vi "write to fifo.vi"(0 "5785_2_x_1600MHz in":refnum<class "5785_2_x_1600MHz.lvclass">, 11 "error in (no error)":errorcluster) -> (4 "5785_2_x_1600MHz out":refnum<class "5785_2_x_1600MHz.lvclass">, 6 "done write file":bool=TRUE, 8 "num of pulses sent to the FPGA":u32, 10 "room on fifo":bool=TRUE, 15 "error out":errorcluster)   [LabVIEW 2021, in "5785_2_x_1600MHz.lvclass"]
uses:
  5785_2_x_1600MHz.lvclass
  5785_2_x_1600MHz.lvclass/5785_2_x_1600MHz.ctl
  <vilib>/Utility/error.llb/Error Cluster From Error Code.vi
  <vilib>/rvi/errors/niLvFpgaAdjustHostInterfaceError.vi
  <vilib>/rvi/interface/nirviMethod/nirviMethod.xnode
  <vilib>/FPGAPlugInAG/Dynamic/niLvFpga_WriteFifo_Dynamic.vi
  <vilib>/rvi/errors/niLvFpgaMergeErrorWithErrorCode.vi
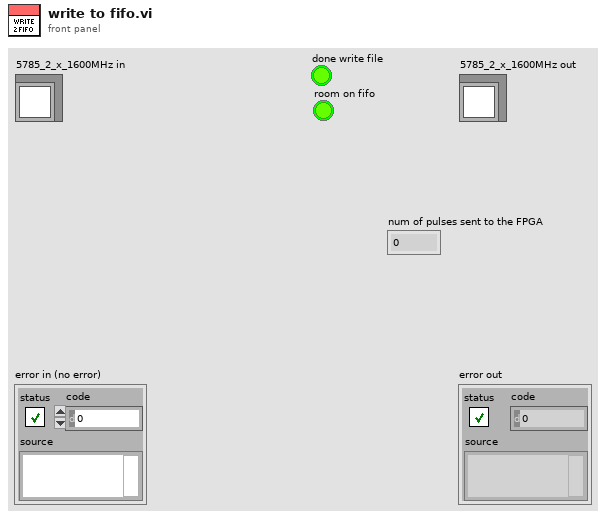
[diagram p1: front panel]
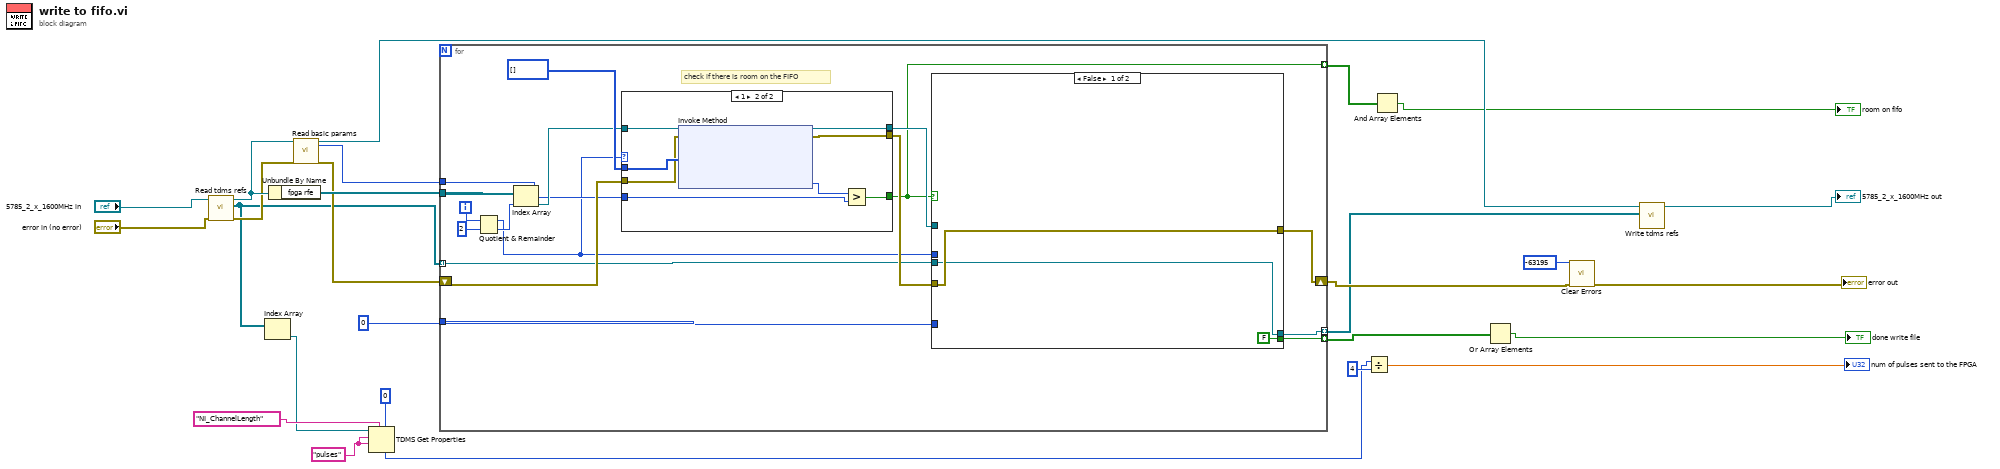
[diagram p0: block diagram]
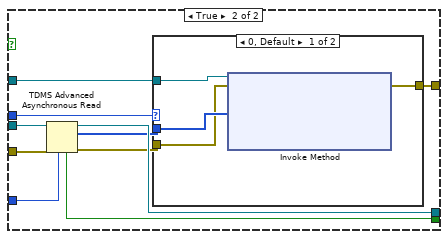
[diagram p2: hidden frame]
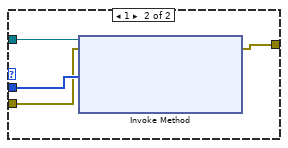
[diagram p3: hidden frame]
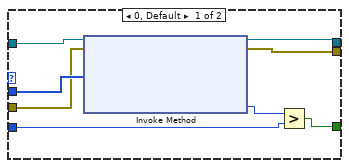
[diagram p4: hidden frame]
diagram:
  w5 = "pulses" ("channel name")
  n1 = call-dynamic "Read tdms refs.vi"("error in (no error)"="error in (no error)", "device_type in"="5785_2_x_1600MHz in") -> ("error out"=w15:errorcluster, "tdms refs"=w3:refnum<k34>[], "device_type out"=w17:refnum<class "5785_2_x_1600MHz.lvclass">)  [unwired: 7 in]
  n2 = Index Array(array=w3) -> (element=w2:refnum<k34>)  [unwired: 1 in]
  n3 = Unbundle By Name(w17) -> ("fpga rfe"=w23:refnum<k20>[])
  n4 = call-dynamic "Read basic params.vi"("device_type in"=w17, "error in (no error)"=w15) -> ("device_type out"=w16:refnum<class "5785_2_x_1600MHz.lvclass">, "buffer size"=w19:u32, "error out"=w14:errorcluster)  [unwired: 12 in, 3 out]
  n5 = TDMS Get Properties(5:u64 0, 7:"NI_ChannelLength" ("property name"), 9:w5, 10:w5, 11:w2) -> (4:w4:u64)  [unwired: 1 in, 5 out]
  n6 = for {
    tunnel: w3 -> [w27] mode=indexing
    tunnel: w23 -> [w43]
    tunnel: u64 0 ("type") -> [w40]
    tunnel: [w39] -> w24 mode=indexing
    tunnel: [w38] -> w18 mode=indexing
    shift-right: [w37] -> w21
    shift-left: w14 -> [w35]
    tunnel: w19 -> [w33]
    tunnel: [w30] -> w20 mode=indexing
    i -> [w28]
    # "check if there is room on the FIFO"
    n7 = Quotient & Remainder(x=w28, y=2) -> (x-y*floor(x/y)=w29:i32, floor(x/y)=w41:i32)
    n8 = Index Array(array=w43, index=w41) -> (element=w34:refnum<k20>)
    n9 = case shown="1" w29 {
      tunnel: w34 -> [w72 w80]
      tunnel: u64[] [] -> [w71 w79]
      tunnel: w35 -> [w70 w78]
      tunnel: [w69 w77] -> w32
      tunnel: w33 -> [w65 w73]
      tunnel: [w67 w75] -> w30
      tunnel: [w66 w74] -> w31
      frame 0, Default {
        n10 = xnode "Invoke Method"("FPGA VI Reference In"=w72, "error in"=w70, "Data"=w71) -> ("FPGA VI Reference Out"=w66:refnum<k20>, "error out"=w69:errorcluster, "Empty Elements Remaining"=w68:u32)  [unwired: 1 in]
        n11 = Greater?(x=w68, y=w65) -> (0:w67:bool)
      }
      frame 1 {
        n12 = xnode "Invoke Method"("FPGA VI Reference In"=w80, "error in"=w78, "Data"=w79) -> ("FPGA VI Reference Out"=w74:refnum<k20>, "error out"=w77:errorcluster, "Empty Elements Remaining"=w76:u32)  [unwired: 1 in]
        n13 = Greater?(x=w76, y=w73) -> (0:w75:bool)
      }
    }
    n14 = case shown="False" w30 {
      tunnel: w27 -> [w44 w47]
      tunnel: w29 -> [_ w56]
      tunnel: w40 -> [_ w55]
      tunnel: [FALSE ("read process finished?") w54] -> w39
      tunnel: [w44 w53] -> w38
      tunnel: [w46 w51] -> w37
      tunnel: w32 -> [w46 w49]
      tunnel: w31 -> [_ w48]
      frame False {
      }
      frame True {
        n15 = TDMS Advanced Asynchronous Read(6:w55, 8:w49, 11:w47) -> (0:w52:errorcluster, 2:w50:u64[], 3:w53:refnum<k34>, 4:w54:bool)
        n16 = case shown="0, Default" w56 {
          tunnel: w48 -> [w60 w64]
          tunnel: w50 -> [w59 w63]
          tunnel: w52 -> [w58 w62]
          tunnel: [w57 w61] -> w51
          frame 0, Default {
            n17 = xnode "Invoke Method"("FPGA VI Reference In"=w60, "error in"=w58, "Data"=w59) -> ("error out"=w57:errorcluster)  [unwired: 1 in, 2 out]
          }
          frame 1 {
            n18 = xnode "Invoke Method"("FPGA VI Reference In"=w64, "error in"=w62, "Data"=w63) -> ("error out"=w61:errorcluster)  [unwired: 1 in, 2 out]
          }
        }
      }
    }
  }
  n19 = Divide(x=w4, y=4) -> (x/y=→"num of pulses sent to the FPGA":dbl)
  n20 = And Array Elements(Boolean array=w20) -> (logical AND=→"room on fifo":bool)
  n21 = Or Array Elements(Boolean array=w24) -> (logical OR=→"done write file":bool)
  n22 = call <vilib>:"Clear Errors.vi"("error in (no error)"=w21, "specific error code to clear (0: all)"=-63195) -> ("error out"=→"error out":errorcluster)  [unwired: 4 in, 1 out]
  n23 = call-dynamic "Write tdms refs.vi"("tdms refs"=w18, "device_type in"=w16) -> ("device_type out"=→"5785_2_x_1600MHz out":refnum<class "5785_2_x_1600MHz.lvclass">)  [unwired: 8 in, 1 out]
